vi "build.iso8601.vi"(11 "Time Series Name":string) -> (3 "ts.iso8601 out":refnum<class "ts.iso8601.lvclass">)   [LabVIEW 2020, in "ts.iso8601.lvclass"]
uses:
  ts.iso8601.lvclass
  C:/code/labview-client/lv_src/timestampMetadata/timestampMetadata.lvclass
  timestampMetadata/timestampMetadata.lvclass/timestampMetadata.ctl
  timestampMetadata/seriesName.set.vi
  ts.iso8601.lvclass/ts.iso8601.ctl
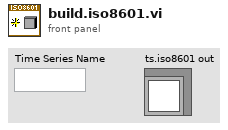
[diagram p1: front panel]
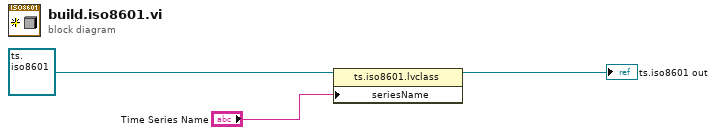
[diagram p0: block diagram]
diagram:
  n1 = property class="ts.iso8601.lvclass"(reference=refnum<class "ts.iso8601.lvclass"> refnum ("ts.iso8601 in"), "seriesName"="Time Series Name") -> (reference out=→"ts.iso8601 out":refnum<class "ts.iso8601.lvclass">)  [unwired: 1 in, 1 out]
